vi "Query Bin Format.vi"(0 "RedPitaya connection in":refnum<k5>, 5 "SCPI Query":string="ACQ:BUF:SIZE?", 9 "timeout ms (2000)":i32=2000, 11 "error in":errorcluster) -> (4 "RedPitaya connection out":refnum<k5>, 6 "data out":string, 15 "error out":errorcluster)   [LabVIEW 2021, in "RedPitaya.lvlib"]
uses:
  RedPitaya.lvlib
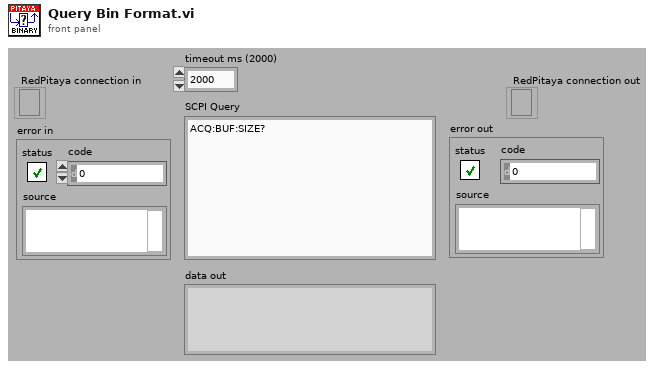
[diagram p1: front panel]
types:
  T1 = enum16{"Standard", "Buffered", "CRLF", "Immediate"}
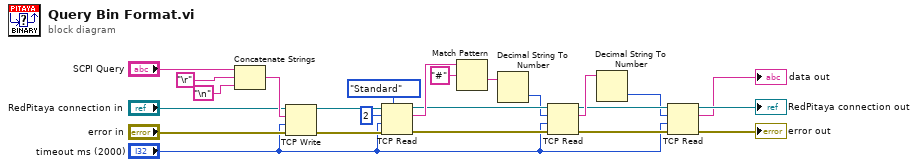
[diagram p0: block diagram]
diagram:
  n1 = Concatenate Strings("SCPI Query", "\r", "\n") -> (w19:string)
  n2 = TCP Write(connection ID="RedPitaya connection in", data in=w19, error in (no error)="error in", 9:"timeout ms (2000)") -> (connection ID out=w24:refnum<k5>, error out=w23:errorcluster)  [unwired: 1 out]
  n3 = TCP Read(connection ID=w24, bytes to read=2, error in (no error)=w23, 7:T1."Standard" ("mode (standard)"), 9:"timeout ms (2000)") -> (connection ID out=w10:refnum<k5>, data out=w14:string, error out=w11:errorcluster)
  n4 = Match Pattern(string=w14, regular expression="#") -> (after substring=w12:string)  [unwired: 1 in, 3 out]
  n5 = Decimal String To Number(string=w12) -> (number=w9:i32)  [unwired: 2 in, 1 out]
  n6 = TCP Read(connection ID=w10, bytes to read=w9, error in (no error)=w11, 9:"timeout ms (2000)") -> (connection ID out=w5:refnum<k5>, data out=w8:string, error out=w7:errorcluster)  [unwired: 1 in]
  n7 = Decimal String To Number(string=w8) -> (number=w3:i32)  [unwired: 2 in, 1 out]
  n8 = TCP Read(connection ID=w5, bytes to read=w3, error in (no error)=w7, 9:"timeout ms (2000)") -> (connection ID out=→"RedPitaya connection out":refnum<k5>, data out=→"data out":string, error out=→"error out":errorcluster)  [unwired: 1 in]
